vi "XML Reader Get Section Elements.vi"(8 "error in":errorcluster, 11 "XML Reader In":T1) -> (0 "error out":errorcluster, 2 "Element Names":string[](array[string]), 3 "XML Reader Out":T1)   [LabVIEW 2017, in "Pathloss XML Reader.lvlib"]
uses:
  Pathloss XML Reader.lvlib
  Controls/XML Reader Data Ref.ctl
  Controls/XML Reader Data.ctl
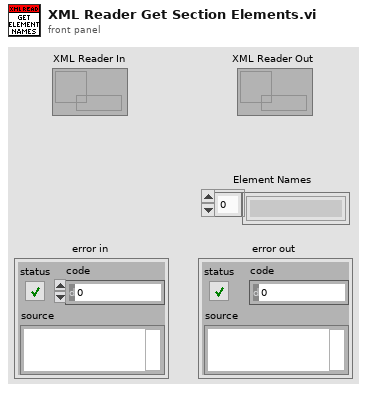
[diagram p1: front panel]
types:
  T1 = typedef "Pathloss XML Reader.lvlib/XML Reader Data Ref.ctl" = refnum<data-value>
  T2 = typedef "Pathloss XML Reader.lvlib/XML Reader Data.ctl" = cluster{"Remaining XML":string, "Section Name Stack":string[], "Section Stack":string[]}
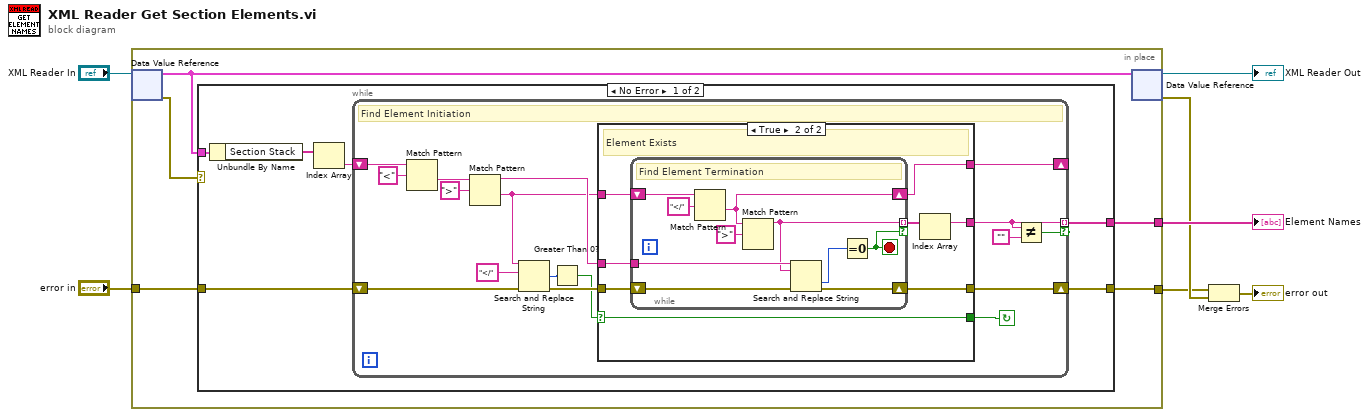
[diagram p0: block diagram]
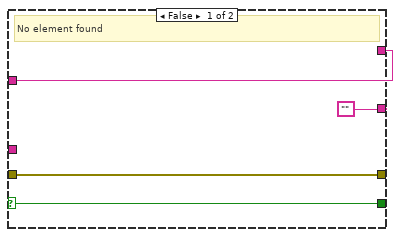
[diagram p2: hidden frame]
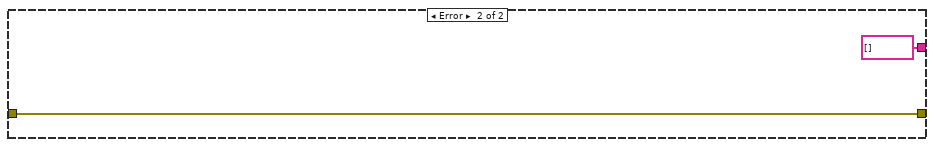
[diagram p3: hidden frame]
diagram:
  n1 = in-place {
    in-place-border: [w11] -> w6
    in-place-border: [w10] -> w2
    in-place-border: "error in" -> [w8]
    n2 = in-place-dvr #1("XML Reader In") -> (w12:T2, w9:errorcluster)
    n3 = case shown="No Error" w9 {
      tunnel: w12 -> [w17 _]
      tunnel: [w16 string[] []] -> w11
      tunnel: [w14 w59] -> w10
      tunnel: w8 -> [w13 w59]
      frame No Error {
        n4 = Unbundle By Name(w17) -> ("Section Stack"=w18:string[])
        n5 = Index Array(array=w18) -> (element=w15:string)  [unwired: 1 in]
        n6 = while {
          tunnel: [w23] -> w16 mode=indexing if=w24
          shift-right: [w31] -> _
          shift-left: w15 -> [w35]
          shift-right: [w21] -> w14
          shift-left: w13 -> [w20]
          stop <- w19 continue-if-true
          # "Find Element Initiation"
          n7 = Match Pattern(string=w35, regular expression="<") -> (after substring=w33:string)  [unwired: 1 in, 3 out]
          n8 = Match Pattern(string=w33, regular expression=">") -> (before substring=w30:string, after substring=w29:string)  [unwired: 1 in, 2 out]
          n9 = Search and Replace String(input string=w29, search string="</" ("regular expression"), error in=w20) -> (number of replacements=w27:i32, error out=w28:errorcluster)  [unwired: 5 in, 2 out]
          n10 = Greater Than 0?(x=w27) -> (x > 0?=w25:bool)
          n11 = case shown="True" w25 {
            selector: w25 -> [w36 w40]
            tunnel: w29 -> [w39 w46]
            tunnel: w30 -> [_ w45]
            tunnel: [w39 w44] -> w31
            tunnel: ["" w43] -> w23
            tunnel: w28 -> [w37 w42]
            tunnel: [w37 w41] -> w21
            tunnel: [w36 w40] -> w19
            frame False {
              # "No element found"
            }
            frame True {
              # "Element Exists"
              n12 = while {
                shift-right: [w55] -> w44
                shift-left: w46 -> [w56]
                tunnel: [w53] -> w47 mode=indexing if=w48
                tunnel: w45 -> [w54]
                shift-right: [w50] -> w41
                shift-left: w42 -> [w52]
                stop <- w48 stop-if-true
                # "Find Element Termination"
                n13 = Match Pattern(string=w56, regular expression="</") -> (after substring=w55:string)  [unwired: 1 in, 3 out]
                n14 = Match Pattern(string=w55, regular expression=">") -> (before substring=w53:string)  [unwired: 1 in, 3 out]
                n15 = Search and Replace String(input string=w54, search string=w53, error in=w52) -> (offset past replacement=w49:i32, error out=w50:errorcluster)  [unwired: 5 in, 2 out]
                n16 = Equal To 0?(x=w49) -> (x = 0?=w48:bool)
              }
              n17 = Index Array(array=w47) -> (element=w43:string)  [unwired: 1 in]
            }
          }
          n18 = Not Equal?(x=w23, y="") -> (x != y?=w24:bool)
        }
      }
      frame Error {
      }
    }
    n19 = in-place-dvr #1(w12) -> (→"XML Reader Out":T1, w3:errorcluster)
  }
  "Element Names" <- w6
  n20 = Merge Errors(w2, w3) -> (→"error out":errorcluster)
